vi "Table, Set Cell Color.vi"(4 "Enable (T)":bool=TRUE, 5 "BGColor Default":u32(colorbox)=16448250, 6 "BGColor Enabled":u32(colorbox)=16744640, 7 "error in":errorcluster, 8 "col (0)":i32, 9 "row (0)":i32, 10 "Tbl Refnum":refnum<vi>) -> (0 "error out":errorcluster, 1 "col+1":i32, 2 "row+1":i32, 3 "Tbl Refnum out":refnum<vi>)   [LabVIEW 2010]
doc: "Sets the active table cell and changes its background color attribute."
uses:
  <vilib>/Utility/miscctls.llb/LVRowAndColumnTypeDef.ctl
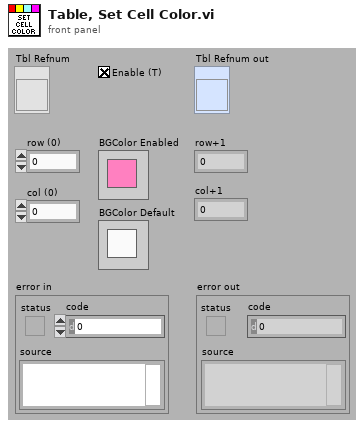
[diagram p1: front panel]
types:
  T1 = typedef "LVRowAndColumnTypeDef.ctl" = cluster{"Row":i32, "Column":i32}
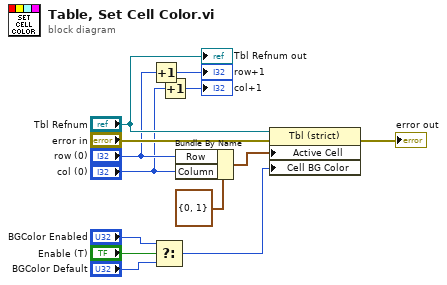
[diagram p0: block diagram]
diagram:
  n1 = Increment(x="row (0)") -> (x+1=→"row+1":i32)
  n2 = Select(t="BGColor Enabled", s="Enable (T)", f="BGColor Default") -> (s? t:f=w5:u32)
  n3 = Increment(x="col (0)") -> (x+1=→"col+1":i32)
  n4 = Bundle By Name(cluster=T1 {"Row"=0, "Column"=1} ("Selection Start 2"), "Row"="row (0)", "Column"="col (0)") -> (w10:T1)
  n5 = property class="Tbl (strict)"(reference="Tbl Refnum", error in="error in", "Active Cell"=w10, "Cell BG Color"=w5) -> (error out=→"error out":errorcluster)  [unwired: 1 out]
  "Tbl Refnum out" <- "Tbl Refnum"
